vi "ni_move_backlash_loop.vi"(6 "Axis enable":bool[](array[boolean])=[TRUE, TRUE, TRUE, TRUE], 8 "error in":errorcluster, 9 "Axis positions":dbl[](array[numeric]), 11 "Absolute":bool=TRUE) -> (0 "error out":errorcluster, 1 "Final axis errors":i32[](array[numeric]))   [LabVIEW 2014]
panel:
  out "Retry count":i32
  in  "Max error":i32=3
  # "Loop doing backlash move until the error is small enough."
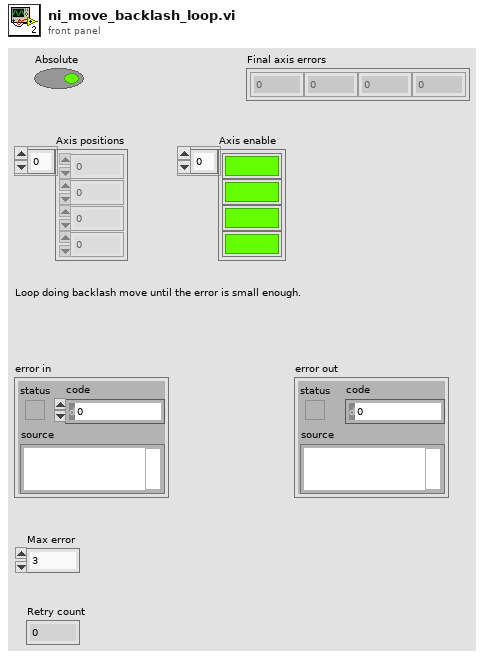
[diagram p1: front panel]
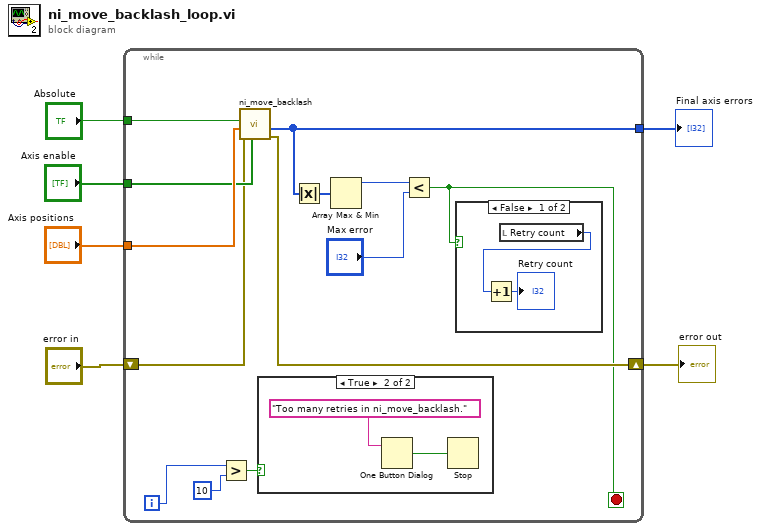
[diagram p0: block diagram]
diagram:
  n1 = while {
    tunnel: "Absolute" -> [w19]
    tunnel: "Axis positions" -> [w18]
    tunnel: "Axis enable" -> [w17]
    tunnel: [w14] -> w1
    shift-right: [w15] -> w2
    shift-left: "error in" -> [w16]
    i -> [w10]
    stop <- w7 stop-if-true
    n2 = Greater?(x=w10, y=10) -> (0:w8:bool)
    n3 = call "ni_move_backlash.vi"("Axis enable"=w17, "error in"=w16, "Axis positions"=w18, "Absolute"=w19) -> ("error out"=w15:errorcluster, "Final axis errors"=w14:i32[])  [unwired: 6 in]
    n4 = case shown="True" w8 {
      frame False {
      }
      frame True {
        n5 = One Button Dialog(message="Too many retries in ni_move_backlash.") -> (true=w22:bool)  [unwired: 1 in]
        n6 = Stop(stop? (T)=w22) -> ()
      }
    }
    n7 = Absolute Value(x=w14) -> (abs(x)=w13:i32[])
    n8 = Array Max & Min(array=w13) -> (max value=w12:i32)  [unwired: 3 out]
    n9 = Less?(x=w12, y="Max error") -> (x < y?=w7:bool)
    n10 = case shown="False" w7 {
      frame False {
        n11 = local read "Retry count"() -> (w20:i32)
        n12 = Increment(x=w20) -> (x+1=→"Retry count":i32)
      }
      frame True {
      }
    }
  }
  "error out" <- w2
  "Final axis errors" <- w1
